vi "Control Data - When Set Explicity - Returns Configured Value.vi"() -> ()   [LabVIEW 2017, in "Test Case.Tests.lvlib"]
uses:
  Test Case.Tests.lvlib
  Test Case/Test Case.lvclass
  ControlData.ctl
  Test Case/Test Case.lvclass/Test Case.ctl
  0e7b8b09-8152-473b-abc1-b62715c3083e.vi
  Test Case/Set Control Data.vi
  Test Case/Get Control Data.vi
  Constraint/IsEqual/Create.vi
  Constraint/IsEqual/IsEqual.lvclass
panel:
  out "error out":errorcluster
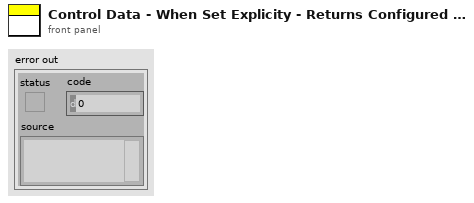
[diagram p1: front panel]
types:
  T1 = typedef "ControlData.ctl" = cluster{"Name":string, "Data":variant}
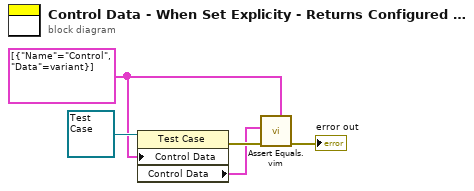
[diagram p0: block diagram]
diagram:
  w1 = T1[] [{"Name"="Control", "Data"=variant}] ("Control Data")
  n1 = property class="Test Case"(reference=refnum<class "Test Case.lvclass"> refnum ("Test Case"), "Control Data"=w1) -> (error out=w4:errorcluster, "Control Data"=w2:T1[])  [unwired: 1 in, 1 out]
  n2 = call "Assert Equals.vim"("Expected"=w1, "error in (no error)"=w4, "Actual"=w2) -> ("error out"=→"error out":errorcluster)  [unwired: 8 in]
